vi "_TEST_ObjCacher4.vi"() -> ()   [LabVIEW 2017]
uses:
  a0d92a37-707b-4f1b-ae9e-3f3d2df0a26e.vi
  4c2e9e81-8d0f-4bb8-9ac8-1d8b5cfdf069.vi
  32b00bf8-5319-4366-93b2-8f71969c86e7.vi
  8edb914a-d4d2-48da-ab29-76f01e13c48e.vi
  b57aafa9-e656-4cc4-a035-61984da44bc1.vi
  bbab33be-48d8-430b-b6cf-34be62a53e80.vi
  ebdc37cc-0830-46f4-b657-e5fc30bcdac4.vi
  131bd1c9-94c7-4ab5-ad2c-58bc16c1b027.vi
  a0d92a37-707b-4f1b-ae9e-3f3d2df0a26e.vi/bbfb678d-0dd1-42b5-aa34-bcbb9bc47f58.vi
  4c2e9e81-8d0f-4bb8-9ac8-1d8b5cfdf069.vi/bbfb678d-0dd1-42b5-aa34-bcbb9bc47f58.vi
  32b00bf8-5319-4366-93b2-8f71969c86e7.vi/bbfb678d-0dd1-42b5-aa34-bcbb9bc47f58.vi
  8edb914a-d4d2-48da-ab29-76f01e13c48e.vi/eadabf24-ff94-4685-a64b-5d14bb58e900.vi
  8edb914a-d4d2-48da-ab29-76f01e13c48e.vi/6b63a7d9-2d15-4471-a336-59ea210d0e91.vi
  8edb914a-d4d2-48da-ab29-76f01e13c48e.vi/f4546358-8284-4e82-84b2-162a8f6e8dde.vi
  b57aafa9-e656-4cc4-a035-61984da44bc1.vi/f4b9e50f-b6c7-4723-8812-5e25554064bb.vi
  bbab33be-48d8-430b-b6cf-34be62a53e80.vi/f4b9e50f-b6c7-4723-8812-5e25554064bb.vi
  ebdc37cc-0830-46f4-b657-e5fc30bcdac4.vi/f4b9e50f-b6c7-4723-8812-5e25554064bb.vi
  131bd1c9-94c7-4ab5-ad2c-58bc16c1b027.vi/f4b9e50f-b6c7-4723-8812-5e25554064bb.vi
  8edb914a-d4d2-48da-ab29-76f01e13c48e.vi/f4546358-8284-4e82-84b2-162a8f6e8dde.vi/db6e846d-7ffa-4d7b-a5d8-6f40a6ea3e17.vi
  Data/_support/Get DataType Description String.vi
  _support/Resource.vi
  2f2337d1-6c97-4f54-a788-925851aa52e2.vi
  fc461ce2-cdf9-4eb3-a08c-dbf1edfd7f95.vi
  70c9e2fc-2fea-4f8f-8306-cfcbe3863a72.vi
  03c23b7a-9b90-40d1-a4fc-a0f708b12f7b.vi
  83e467ab-086d-413c-8552-dff3e4b96e82.vi
  75ce0f79-ffd3-4117-ae33-183ac051c13f.vi
panel:
  out "cacher":variant
  out "x-y 3":u32[](array[numeric])=[100, 392, 882, 1568, 2470, 3549, 4854, 6384, 8469, 10070]
  out "XY Graph":cluster{"Array 3":i32[], "x-y 2":u32[]}(graph)={"Array 3"=[100, 200, 300, 400, 500, 600, 700, 800, 900, 1000], "x-y 2"=[100, 392, 882, 1568, 2470, 3549, 4854, 6384, 8469, 10070]}
  in  "Array 3":i32[](array[numeric])=[100, 200, 300, 400, 500, 600, 700, 800, 900, 1000]
  out "x-y 2":u32[](array[numeric])=[100, 392, 882, 1568, 2470, 3549, 4854, 6384, 8469, 10070]
  out "Array 2":u32[](array[numeric])=[3621, 6, 5, 5, 5, 6, 5, 4, 5, 4]
  out "Array":T1(array[cluster])
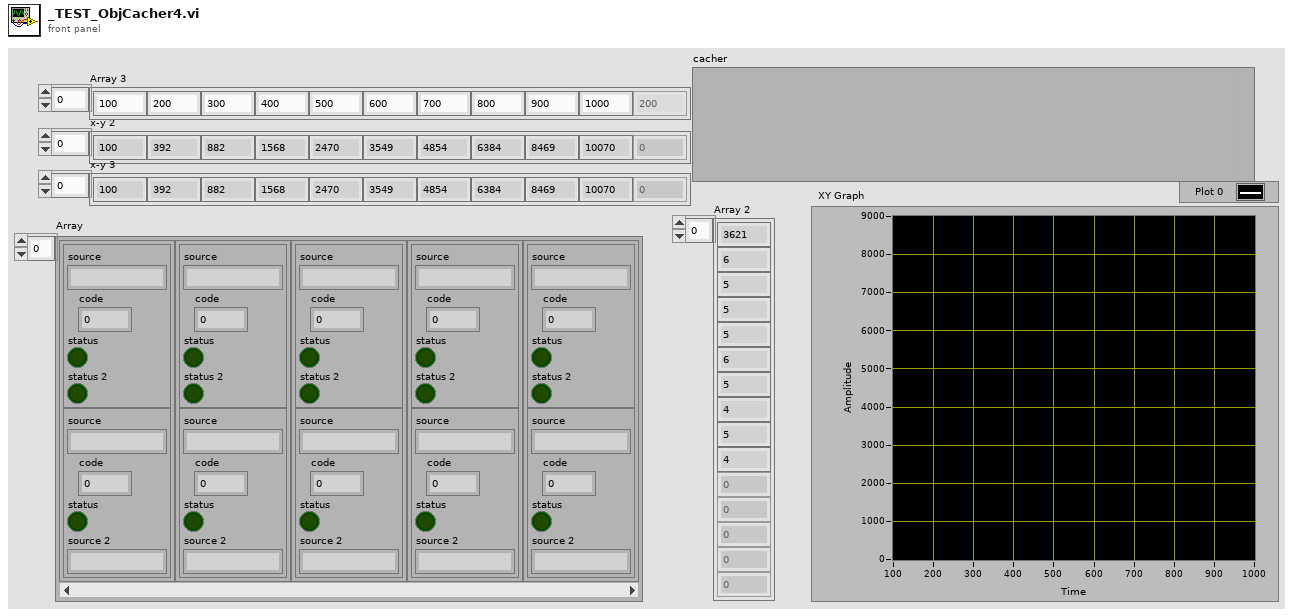
[diagram p1: front panel]
types:
  T1 = cluster{cluster{"source":string, "code":i32, "status":bool, "status 2":bool}, cluster{"source":string, "code":i32, "status":bool, "source 2":string}}[]
  T2 = cluster{cluster{"source":string, "code":i32, "status":bool, "status 2":bool}, cluster{"source":string, "code":i32, "status":bool, "source 2":string}}
  T3 = cluster{"source":string, "code":i32, "status":bool, "source 2":string}
  T4 = cluster{"source":string, "code":i32, "status":bool, "status 2":bool}
  T5 = cluster{"source":string, "code":i32, "status":bool}
  T6 = cluster{"source":string, "code":i32, "status":bool}[]
  T7 = cluster{"source":string, "code":i32, "status":bool, "status 2":bool}[]
  T8 = cluster{"source":string, "code":i32, "status":bool, "source 2":string}[]
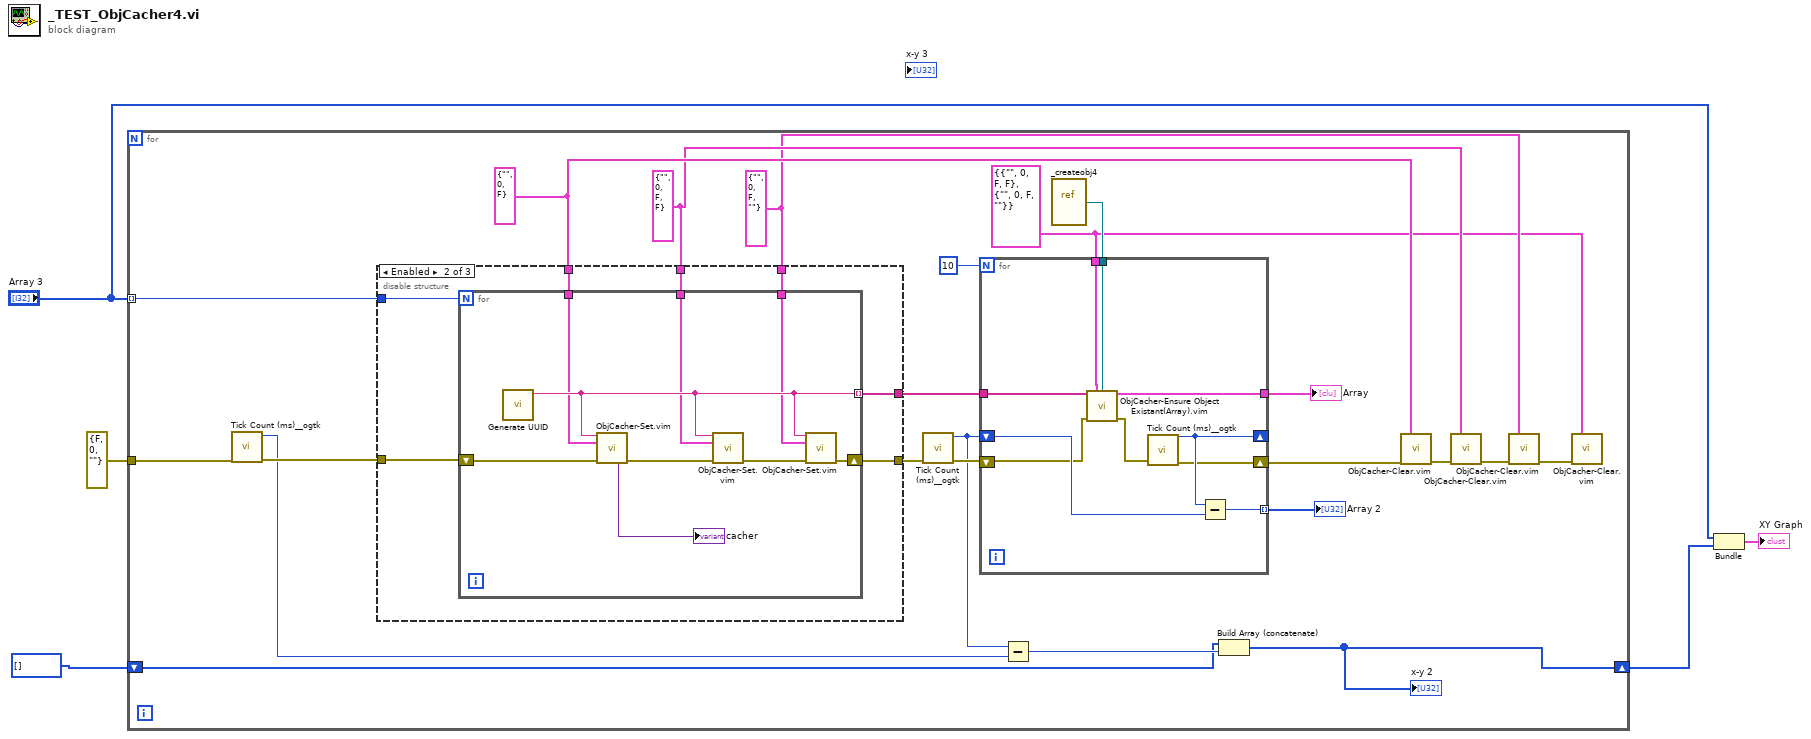
[diagram p0: block diagram]
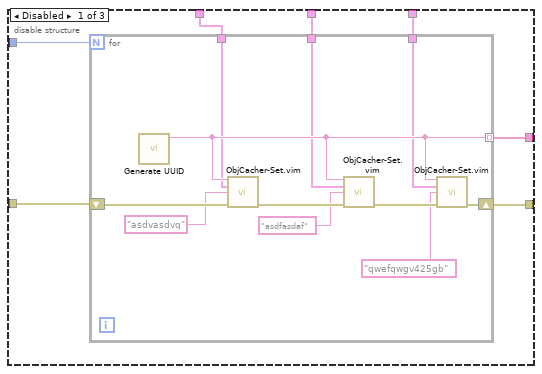
[diagram p2: hidden frame]
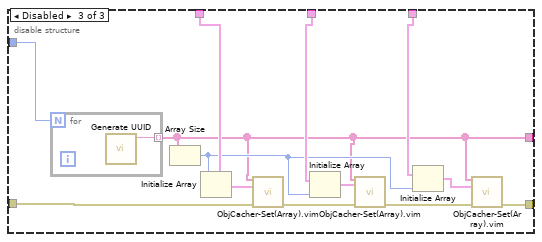
[diagram p3: hidden frame]
diagram:
  n1 = for {
    tunnel: "Array 3" -> [w25] mode=indexing
    shift-right: [w15] -> w4
    shift-left: u32[] [] ("x-y") -> [w16]
    tunnel: errorcluster {"status"=FALSE, "code"=0, "source"=""} ("error out") -> [w6]
    w10 = T2 {{"source"="", "code"=0, "status"=FALSE, "status 2"=FALSE}, {"source"="", "code"=0, "status"=FALSE, "source 2"=""}}
    w11 = T3 {"source"="", "code"=0, "status"=FALSE, "source 2"=""}
    w12 = T4 {"source"="", "code"=0, "status"=FALSE, "status 2"=FALSE}
    w13 = T5 {"source"="", "code"=0, "status"=FALSE}
    n2 = call <userlib>:"Tick Count (ms)__ogtk.vi"("error in (no error)"=w6) -> ("error out"=w20:errorcluster, "millisecond timer value"=w18:u32)  [unwired: 9 in]
    n3 = disable-structure shown="Enabled" {
      disable-tunnel: [w35 w53 w63] -> w28
      disable-tunnel: w25 -> [w34 w52 w71]
      disable-tunnel: [w33 w51 w75] -> w23
      disable-tunnel: w20 -> [w32 w50 w74]
      disable-tunnel: w13 -> [w31 w49 w70]
      disable-tunnel: w12 -> [w30 w48 w68]
      disable-tunnel: w11 -> [w29 w47 w66]
      frame Disabled {
        n4 = for {
          N: w34 -> [_]
          tunnel: [w43] -> w35 mode=indexing
          shift-right: [w44] -> w33
          shift-left: w32 -> [w42]
          tunnel: w31 -> [w41]
          tunnel: w30 -> [w40]
          tunnel: w29 -> [w39]
          n5 = call "Generate UUID.vi"() -> ("UUID"=w43:string)  [unwired: 11 in]
          n6 = call "ObjCacher-Set.vim"("Module Name"=w43, "data"=w41, "typeKey(\"\" to use DataTypeDescription)"="asdvasdvq" ("typeKey(\"\" to use DataTypeDescription)"), "error in (no error)"=w42) -> ("error out"=w46:errorcluster)  [unwired: 9 in, 2 out]
          n7 = call "ObjCacher-Set.vim"("Module Name"=w43, "data"=w40, "typeKey(\"\" to use DataTypeDescription)"="asdfasdaf" ("typeKey(\"\" to use DataTypeDescription)"), "error in (no error)"=w46) -> ("error out"=w45:errorcluster)  [unwired: 9 in, 2 out]
          n8 = call "ObjCacher-Set.vim"("Module Name"=w43, "data"=w39, "typeKey(\"\" to use DataTypeDescription)"="qwefqwgv425gb" ("typeKey(\"\" to use DataTypeDescription)"), "error in (no error)"=w45) -> ("error out"=w44:errorcluster)  [unwired: 9 in, 2 out]
        }
      }
      frame Enabled {
        n9 = for {
          N: w52 -> [_]
          tunnel: [w59] -> w53 mode=indexing
          shift-right: [w60] -> w51
          shift-left: w50 -> [w58]
          tunnel: w49 -> [w57]
          tunnel: w48 -> [w56]
          tunnel: w47 -> [w55]
          n10 = call "Generate UUID.vi"() -> ("UUID"=w59:string)  [unwired: 11 in]
          n11 = call "ObjCacher-Set.vim"("Module Name"=w59, "data"=w57, "error in (no error)"=w58) -> ("cacher"=→"cacher":variant, "error out"=w62:errorcluster)  [unwired: 10 in, 1 out]
          n12 = call "ObjCacher-Set.vim"("Module Name"=w59, "data"=w56, "error in (no error)"=w62) -> ("error out"=w61:errorcluster)  [unwired: 10 in, 2 out]
          n13 = call "ObjCacher-Set.vim"("Module Name"=w59, "data"=w55, "error in (no error)"=w61) -> ("error out"=w60:errorcluster)  [unwired: 10 in, 2 out]
        }
      }
      frame Disabled {
        n14 = for {
          N: w71 -> [_]
          tunnel: [w76] -> w63 mode=indexing
          n15 = call "Generate UUID.vi"() -> ("UUID"=w76:string)  [unwired: 11 in]
        }
        n16 = Array Size(array=w63) -> (size(s)=w65:i32)
        n17 = Initialize Array(w70, w65) -> (w69:T6)
        n18 = call "ObjCacher-Set(Array).vim"("Module Name"=w63, "data"=w69, "error in (no error)"=w74) -> ("error out"=w73:errorcluster)  [unwired: 10 in, 2 out]
        n19 = Initialize Array(w68, w65) -> (w67:T7)
        n20 = call "ObjCacher-Set(Array).vim"("Module Name"=w63, "data"=w67, "error in (no error)"=w73) -> ("error out"=w72:errorcluster)  [unwired: 10 in, 2 out]
        n21 = Initialize Array(w66, w65) -> (w64:T8)
        n22 = call "ObjCacher-Set(Array).vim"("Module Name"=w63, "data"=w64, "error in (no error)"=w72) -> ("error out"=w75:errorcluster)  [unwired: 10 in, 2 out]
      }
    }
    n23 = call <userlib>:"Tick Count (ms)__ogtk.vi"("error in (no error)"=w23) -> ("error out"=w22:errorcluster, "millisecond timer value"=w19:u32)  [unwired: 9 in]
    n24 = Subtract(x=w19, y=w18) -> (x-y=w17:u32)
    n25 = vi-ref "_createobj4.vi"() -> (w27:refnum<vi>)
    n26 = for {
      N: 10 -> [_]
      tunnel: w28 -> [w86]
      tunnel: w27 -> [w85]
      tunnel: [w84] -> w26
      shift-right: [w83] -> _
      shift-left: w19 -> [w82]
      tunnel: [w81] -> w21 mode=indexing
      shift-right: [w78] -> w14
      shift-left: w22 -> [w79]
      tunnel: w10 -> [w77]
      n27 = call "ObjCacher-Ensure Object Existant(Array).vim"("Module Name"=w86, "Variant"=w77, "Generator VI Ref"=w85, "error in (no error)"=w79) -> ("Array"=w84:T1, "error out"=w80:errorcluster)  [unwired: 9 in, 1 out]
      n28 = call <userlib>:"Tick Count (ms)__ogtk.vi"("error in (no error)"=w80) -> ("error out"=w78:errorcluster, "millisecond timer value"=w83:u32)  [unwired: 9 in]
      n29 = Subtract(x=w83, y=w82) -> (x-y=w81:u32)
    }
    "Array" <- w26
    "Array 2" <- w21
    n30 = Build Array (concatenate)(w16, w17) -> (w15:u32[])
    "x-y 2" <- w15
    n31 = call "ObjCacher-Clear.vim"("type"=w13, "error in (no error)"=w14) -> ("error out"=w8:errorcluster)  [unwired: 11 in, 2 out]
    n32 = call "ObjCacher-Clear.vim"("type"=w12, "error in (no error)"=w8) -> ("error out"=w9:errorcluster)  [unwired: 11 in, 2 out]
    n33 = call "ObjCacher-Clear.vim"("type"=w11, "error in (no error)"=w9) -> ("error out"=w7:errorcluster)  [unwired: 11 in, 2 out]
    n34 = call "ObjCacher-Clear.vim"("type"=w10, "error in (no error)"=w7) -> ()  [unwired: 11 in, 3 out]
  }
  n35 = Bundle("Array 3"="Array 3", "x-y"=w4) -> (→"XY Graph":cluster{"Array 3":i32[], "x-y":u32[]})  [unwired: 1 in]
